vi "real_web_old.vi"(11 "httpRequestID":u32) -> (3 "httpRequestID out":u32)   [LabVIEW 2011]
uses:
  <vilib>/Utility/file.llb/Write To Spreadsheet File (string).vi
  <vilib>/addons/database/Connection.llb/DB Tools Open Connec (String).vi
  <vilib>/wsapi/NI_WebServices.lvlib
  <vilib>/addons/database/NI_Database_API.lvlib
panel:
  out "error out":errorcluster
  in  "all request variables":path=path "c:/htmlprop.txt"
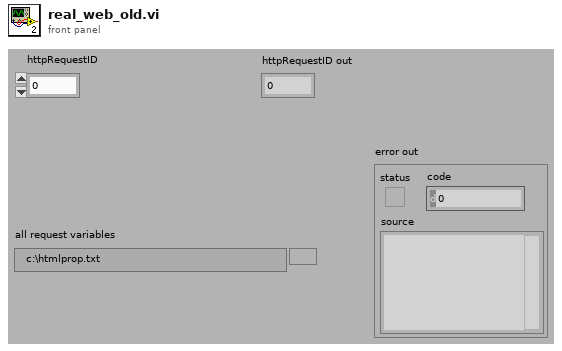
[diagram p1: front panel]
types:
  T1 = typedef "NI_Database_API.lvlib/Conn ObjectReference.ctl" = refnum<k1>
  T2 = cluster{cluster{bool, bool, bool, bool}, cluster{bool, bool, bool, bool}, bool, bool, cluster{"value":string, "value":string}}
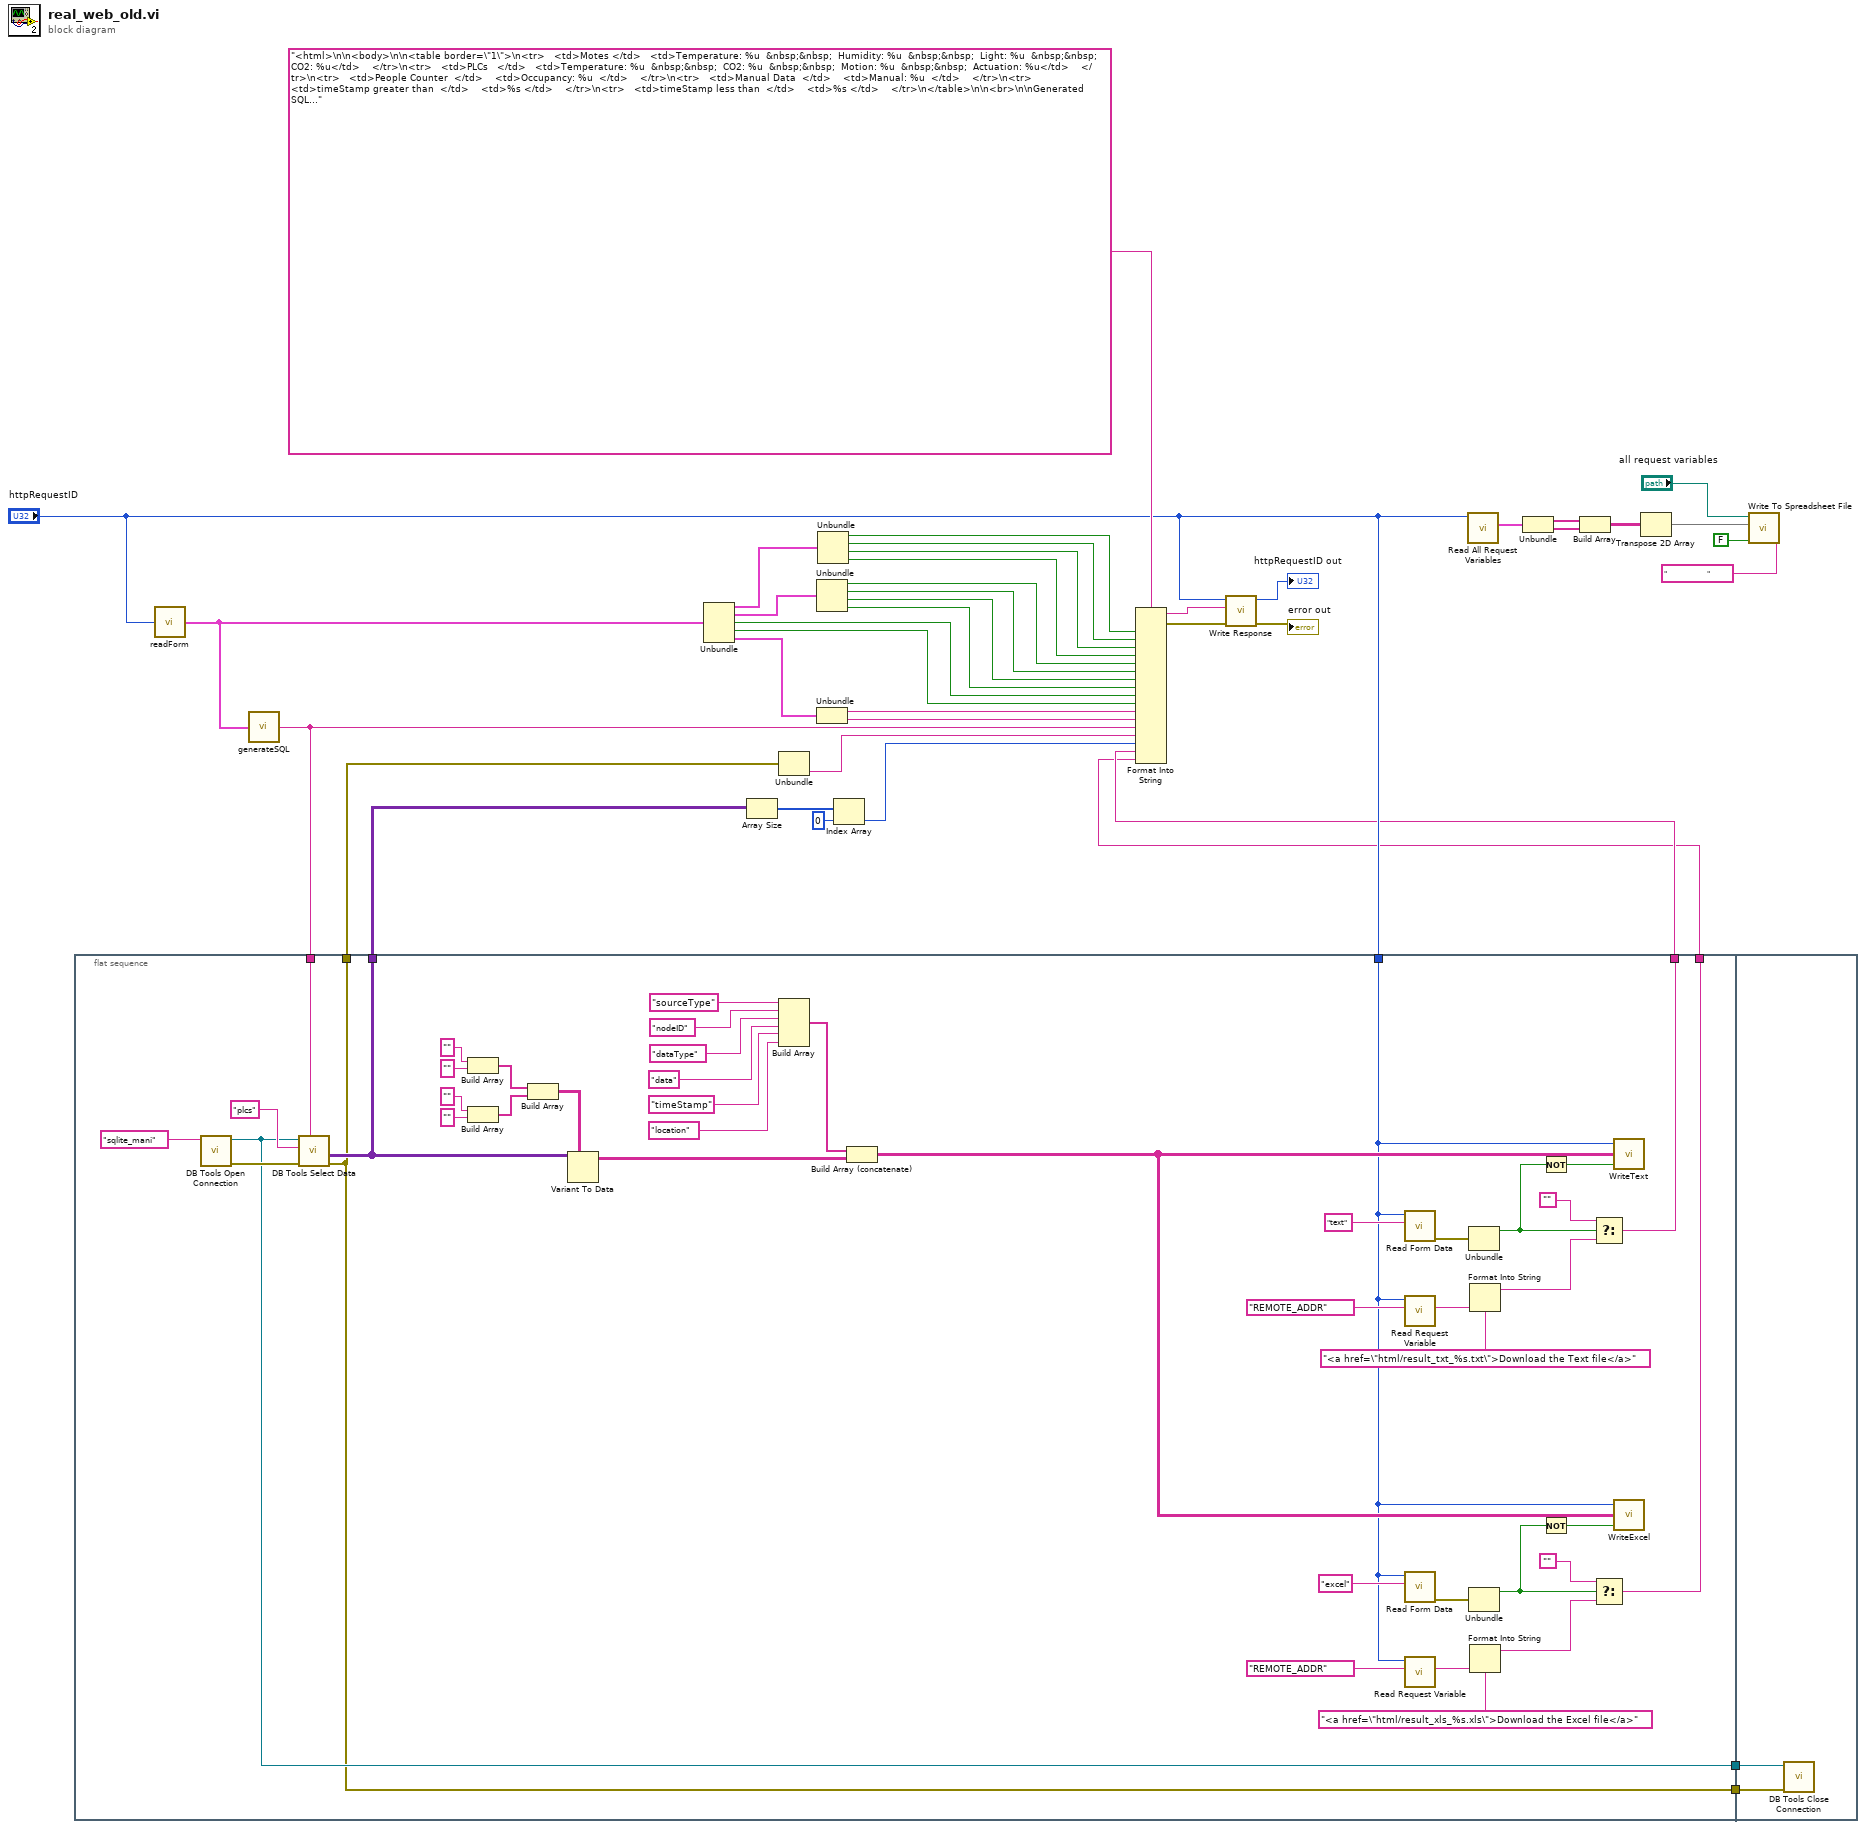
[diagram p0: block diagram]
diagram:
  n1 = flat-sequence {
    tunnel: [w43] -> w41
    tunnel: [w76] -> w32
    tunnel: w2 -> [w67]
    tunnel: "httpRequestID" -> [w47]
    tunnel: [w46] -> w4
    tunnel: [w45] -> w3
    tunnel: [w44] -> w23
    tunnel: [w43] -> w22
    tunnel: w23 -> [w87]
    tunnel: w22 -> [w86]
    frame #0 {
      n2 = call-poly <vilib>:"DB Tools Open Connection.vi"("connection information"="sqlite_mani") -> ("error out"=w85:errorcluster, "connection reference"=w44:T1)  [unwired: 7 in]
      n3 = call <vilib>:"DB Tools Select Data.vi"("condition"=w67, "error in (no error)"=w85, "table"="plcs", "connection reference"=w44) -> ("error out"=w43:errorcluster, "data"=w76:variant[][])  [unwired: 2 in, 1 out]
      n4 = Build Array("", "") -> (w82:string[])
      n5 = Build Array("", "") -> (w83:string[])
      n6 = Build Array(w82, w83) -> (w84:string[][])
      n7 = Variant To Data(type=w84, Variant=w76) -> (data=w75:string[][])  [unwired: 1 in, 1 out]
      n8 = Build Array("sourceType", "nodeID", "dataType", "data", "timeStamp", "location") -> (w68:string[])
      n9 = Build Array (concatenate)(w68, w75) -> (w48:string[][])
      n10 = call <vilib>:"Read Form Data.vi"("key"="text", "httpRequestID"=w47) -> ("error out"=w65:errorcluster)  [unwired: 1 in, 8 out]
      n11 = call <vilib>:"Read Request Variable.vi"("variable name"="REMOTE_ADDR", "httpRequestID"=w47) -> ("value"=w59:string)  [unwired: 7 in, 2 out]
      n12 = call <vilib>:"Read Form Data.vi"("key"="excel", "httpRequestID"=w47) -> ("error out"=w50:errorcluster)  [unwired: 1 in, 8 out]
      n13 = call <vilib>:"Read Request Variable.vi"("variable name"="REMOTE_ADDR", "httpRequestID"=w47) -> ("value"=w56:string)  [unwired: 7 in, 2 out]
      n14 = Unbundle(w65) -> ("status"=w62:bool)  [unwired: 2 out]
      n15 = Unbundle(w50) -> ("status"=w53:bool)  [unwired: 2 out]
      n16 = Format Into String(format string="<a href=\"html/result_txt_%s.txt\">Download the Text file</a>", w59) -> (resulting string=w58:string)  [unwired: 2 in, 1 out]
      n17 = Format Into String(format string="<a href=\"html/result_xls_%s.xls\">Download the Excel file</a>", w56) -> (resulting string=w57:string)  [unwired: 2 in, 1 out]
      n18 = Not(x=w62) -> (.not. x?=w63:bool)
      n19 = Not(x=w53) -> (.not. x?=w52:bool)
      n20 = Select(t="", s=w62, f=w58) -> (s? t:f=w46:string)
      n21 = Select(t="", s=w53, f=w57) -> (s? t:f=w45:string)
      n22 = call "WriteText.vi"("Boolean"=w63, "Input data"=w48, "httpRequestID"=w47) -> ()  [unwired: 1 in]
      n23 = call "WriteExcel.vi"("Boolean"=w52, "input data"=w48, "httpRequestID"=w47) -> ()  [unwired: 1 in]
    }
    frame #1 {
      n24 = call <vilib>:"DB Tools Close Connection.vi"("error in (no error)"=w86, "connection reference"=w87) -> ()  [unwired: 5 in, 1 out]
    }
  }
  n25 = call "readForm.vi"("httpRequestID"="httpRequestID") -> ("output cluster"=w1:T2)
  n26 = call "generateSQL.vi"("input cluster"=w1) -> ("SQL command"=w2:string)
  n27 = Unbundle(w1) -> (w21:cluster{bool, bool, bool, bool}, w20:cluster{bool, bool, bool, bool}, w11:bool, w10:bool, w9:cluster{"value":string, "value":string})
  n28 = Array Size(array=w32) -> (size(s)=w31:i32[])
  n29 = Unbundle(w41) -> ("source"=w6:string)  [unwired: 2 out]
  n30 = Unbundle(w20) -> (w15:bool, w14:bool, w13:bool, w12:bool)
  n31 = Unbundle(w9) -> ("value"=w8:string, "value"=w7:string)
  n32 = Unbundle(w21) -> (w19:bool, w18:bool, w17:bool, w16:bool)
  n33 = Index Array(array=w31, index=0) -> (element=w5:i32)
  n34 = Format Into String(format string="<html>\n\n<body>\n\n<table border=\"1\">\n<tr>   <td>Motes </td>   <td>Temperature: %u  &nbsp;&nbsp;  Humidity: %u  &nbsp;&nbsp;  Light: %u  &nbsp;&nbsp;  CO2: %u</td>    </tr>\n<tr>   <td>PLCs   </td>   <td>Temperature: %u  &nbsp;&nbsp;  CO2: %u  &nbsp;&nbsp;  Motion: %u  &nbsp;&nbsp;  Actuation: %u</td>    </tr>\n<tr>   <td>People Counter  </td>    <td>Occupancy: %u  </td>    </tr>\n<tr>   <td>Manual Data  </td>    <td>Manual: %u  </td>    </tr>\n<tr>   <td>timeStamp greater than  </td>    <td>%s </td>    </tr>\n<tr>   <td>timeStamp less than  </td>    <td>%s </td>    </tr>\n</table>\n\n<br>\n\nGenerated SQL command: %s  <br>\nAccess to database msg:   %s  <br>\nNumber of retrieved records:   %u <br> <br>\n\n%s <br>\n%s <br>\n\n</body>\n\n</html>", w19, w18, w17, w16, w15, w14, w13, w12, w11, w10, w8, w7, w2, w6, w5, w4, w3) -> (resulting string=w29:string, error out=w28:errorcluster)  [unwired: 2 in]
  n35 = call <vilib>:"Write Response.vi"("error in (no error)"=w28, "response string"=w29, "httpRequestID"="httpRequestID") -> ("error out"=→"error out":errorcluster, "httpRequestID out"=→"httpRequestID out":u32)  [unwired: 7 out]
  n36 = call <vilib>:"Read All Request Variables.vi"("httpRequestID"="httpRequestID") -> ("request variables"=w36:cluster{"Key":string[], "Value":string[]})  [unwired: 8 in, 2 out]
  n37 = Unbundle(w36) -> ("Key"=w37:string[], "Value"=w38:string[])
  n38 = Build Array(w37, w38) -> (w39:string[][])
  n39 = Transpose 2D Array(2D array=w39) -> (transposed array=w40:string[][])
  n40 = call-poly <vilib>:"Write To Spreadsheet File.vi"("delimiter (\\t)"="                    ", "append to file? (new file:F)"=FALSE, "2D data"=w40, "file path (dialog if empty)"="all request variables") -> ()  [unwired: 4 in, 1 out]
